vi "Unregister UIMessage Callback.vi"(6 "UIMessage IDs":T1[](array[typedef]), 8 "error in (no error)":errorcluster, 9 "Callback ID":i32, 10 "Callback":T2, 11 "Engine in":refnum<class "Engine.lvclass">) -> (0 "error out":errorcluster, 3 "Engine out":refnum<class "Engine.lvclass">)   [LabVIEW 2020, in "TSnax.lvlib" / "Engine.lvclass"]
uses:
  Engine.lvclass
  Engine.lvclass/Engine.ctl
  UIMsg.ctl
  TSnax.lvlib
  UIMessage Callback.ctl
  UIMessage/UIMessage.lvclass
  <vilib>/Utility/miscctls.llb/LVMapReplaceAction.ctl
  UIMsg Callback VI.ctl
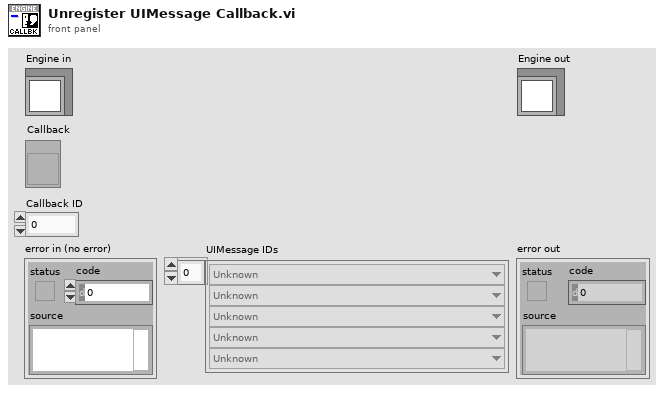
[diagram p1: front panel]
types:
  T1 = typedef "TSnax.lvlib/UIMsg.ctl" = enum16{"Unknown", "BreakOnUserRequest", "BreakOnBreakpoint", "BreakOnRunTimeError", "Trace", "TerminatingExecution", "AbortingExecution", "KillingExecutionThreads", "EndExecution", "ShutDownComplete", "StartExecution", "ProgressPercent", "ProgressText", "StartInteractiveExecution", "EndInteractiveExecution", "TerminatingInteractiveExecution", "TerminationCancelled", "ResumeFromBreak", "StartFileExecution", "EndFileExecution", "ShutDownCancelled", "LocalizationSettingChanged", "OpenWindows", "TileWindows", "CascadeWindows", "ReportChanged", "CloseWindows", "RefreshWindows", "ClientFileChanged", "DisplayReport", "ModelState_Initializing", "ModelState_Waiting", "ModelState_Identified", "ModelState_BeginTesting", "ModelState_TestingComplete", "ModelState_PostProcessingComplete", "ModelState_EnabledStateSet", "ReportLocationChanged", "GotoLocation", "PushUndoItem", "OutputMessages", "TypePaletteFileListChanged", "NonTerminatingThreadsArePreventingTermination", "ModelState_PostProcessing", "ReportCollectionChanged", "RuntimeError"}
  T2 = typedef "TSnax.lvlib/Engine.lvclass/UIMsg Callback VI.ctl" = refnum<vi>
  T3 = typedef "LVMapReplaceAction.ctl" = enum32{"Modify Entry only if found", "Add or Modify Entry", "Delete Entry"}
  T4 = typedef "TSnax.lvlib/Engine.lvclass/UIMessage Callback.ctl" = cluster{"VI":T2, "Owner":refnum<class>, "User Data":variant, "IDs":T1[]}
  T5 = typedef "TSnax.lvlib/Engine.lvclass/UIMessage Callbacks.ctl" = cluster{"Callbacks":T4[], "ID Map":map{T1, i32[]}}
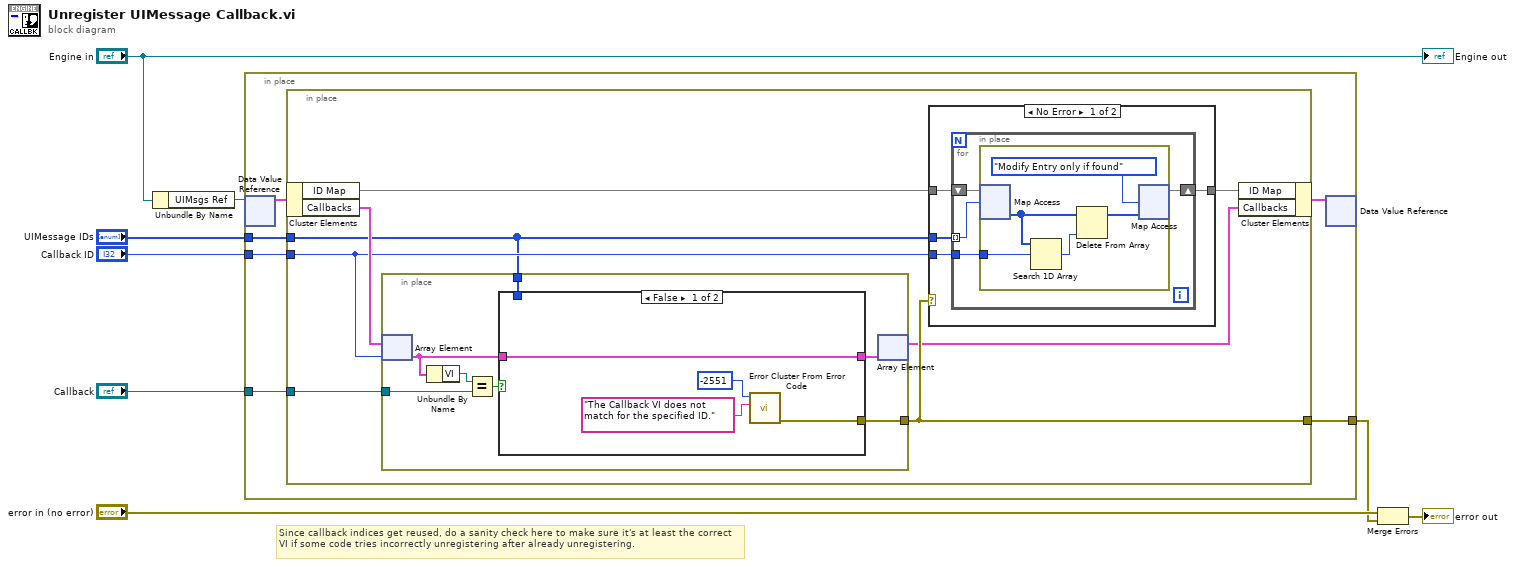
[diagram p0: block diagram]
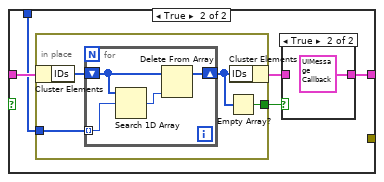
[diagram p3: hidden frame]
diagram:
  # "Since callback indices get reused, do a sanity check here to make sure it's at least the correct VI if some code tries incorrectly unregistering after already unregistering."
  n1 = Unbundle By Name("Engine in") -> ("UIMsgs Ref"=w7:refnum<data-value>)
  n2 = in-place {
    in-place-border: "UIMessage IDs" -> [w12]
    in-place-border: "Callback ID" -> [w11]
    in-place-border: "Callback" -> [w10]
    in-place-border: [w9] -> w1
    n3 = in-place-dvr #1(w7) -> (w14:T5)  [unwired: 1 out]
    n4 = in-place {
      in-place-border: w12 -> [w18]
      in-place-border: w11 -> [w19]
      in-place-border: w10 -> [w20]
      in-place-border: [w22] -> w9
      n5 = in-place-cluster #2(w14) -> ("ID Map"=w16:map{T1, i32[]}, "Callbacks"=w21:T4[])
      n6 = in-place {
        in-place-border: w20 -> [w43]
        in-place-border: w18 -> [w41]
        in-place-border: [w37] -> w22
        n7 = in-place-array #3(w21, w19) -> (w39:T4)
        n8 = Unbundle By Name(w39) -> ("VI"=w42:T2)
        n9 = Equal?(x=w42, y=w43) -> (x = y?=w40:bool)
        n10 = case shown="False" w40 {
          tunnel: w41 -> [_ w51]
          tunnel: w39 -> [w47 w52]
          tunnel: [w47 w48] -> w38
          tunnel: [w44 _] -> w37
          frame False {
            n11 = call <vilib>:"Error Cluster From Error Code.vi"("error message (\"\")"="The Callback VI does not match for the specified ID." ("error message (\"\")"), "error code (0)"=-2551) -> ("error out"=w44:errorcluster)  [unwired: 7 in]
          }
          frame True {
            n12 = in-place {
              in-place-border: w51 -> [w57]
              in-place-border: [w55] -> w49
              n13 = in-place-cluster #4(w52) -> ("IDs"=w58:T1[])
              n14 = for {
                shift-right: [w59] -> w56
                shift-left: w58 -> [w61]
                tunnel: w57 -> [w62] mode=indexing
                n15 = Search 1D Array(1D array=w61, element=w62) -> (index of element=w60:i32)  [unwired: 1 in]
                n16 = Delete From Array(array=w61, index=w60) -> (array with subset deleted=w59:T1[])  [unwired: 1 in, 1 out]
              }
              n17 = Empty Array?(array=w56) -> (empty?=w55:bool)
              n18 = in-place-cluster #4("IDs"=w56) -> (w50:T4)
            }
            n19 = case shown="True" w49 {
              tunnel: w50 -> [w53 _]
              tunnel: [w53 T4 {"VI"=refnum, "Owner"=refnum, "User Data"=variant, "IDs"=[]} ("UIMessage Callback")] -> w48
              frame False {
              }
              frame True {
              }
            }
          }
        }
        n20 = in-place-array #3(w38) -> (w17:T4[])  [unwired: 1 out]
      }
      n21 = case shown="No Error" w22 {
        tunnel: w19 -> [w23 _]
        tunnel: w18 -> [w24 _]
        tunnel: w16 -> [w26 w36]
        tunnel: [w25 w36] -> w15
        frame No Error {
          n22 = for {
            shift-right: [w29] -> w25
            shift-left: w26 -> [w30]
            tunnel: w24 -> [w28] mode=indexing
            tunnel: w23 -> [w27]
            n23 = in-place {
              in-place-border: w27 -> [w34]
              n24 = in-place-map #5(w30, w28) -> (w33:i32[])  [unwired: 1 in, 1 out]
              n25 = Search 1D Array(1D array=w33, element=w34) -> (index of element=w35:i32)  [unwired: 1 in]
              n26 = Delete From Array(array=w33, index=w35) -> (array with subset deleted=w32:i32[])  [unwired: 1 in, 1 out]
              n27 = in-place-map #5(w32, LVMapReplaceAction."Modify Entry only if found" ("action")) -> (w29:map{T1, i32[]})  [unwired: 2 out]
            }
          }
        }
        frame Error {
        }
      }
      n28 = in-place-cluster #2("ID Map"=w15, "Callbacks"=w17) -> (w13:T5)
    }
    n29 = in-place-dvr #1(w13) -> ()  [unwired: 2 out]
  }
  n30 = Merge Errors("error in (no error)", w1) -> (→"error out":errorcluster)
  "Engine out" <- "Engine in"
